vi "Color Map.vi"() -> ()   [LabVIEW 2014]
uses:
  <vilib>/picture/picture.llb/Draw 8-Bit Pixmap.vi
panel:
  out "new picture":picture
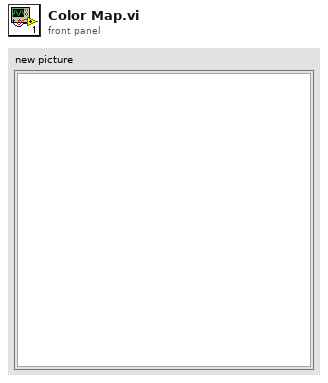
[diagram p1: front panel]
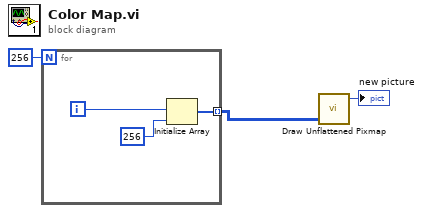
[diagram p0: block diagram]
diagram:
  n1 = for {
    N: 256 -> [_]
    tunnel: [w4] -> w2 mode=indexing
    i -> [w5]
    n2 = Initialize Array(w5, 256 ("dimension size")) -> (w4:i32[])
  }
  n3 = call-poly <vilib>:"Draw Unflattened Pixmap.vi"("data"=w2) -> ("new picture"=→"new picture":picture)  [unwired: 8 in]
